vi "GetVarfromREPL.vi"(8 "error in (no error)":errorcluster, 10 "Command":string, 11 "Server":path) -> (0 "error out":errorcluster, 2 "reply":string)   [LabVIEW 2020]
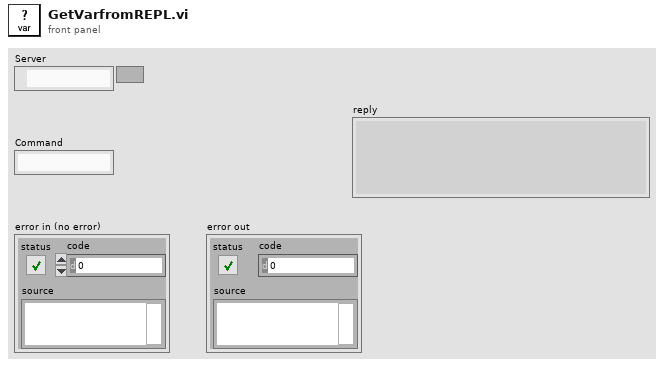
[diagram p1: front panel]
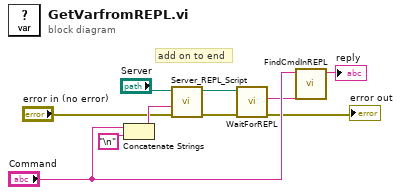
[diagram p0: block diagram]
diagram:
  # "add on to end"
  n1 = Concatenate Strings("Command", "\n") -> (w3:string)
  n2 = call "Server_REPL_Script.vi"("error in (no error)"="error in (no error)", "Code"=w3, "Server"="Server") -> ("error out"=w2:errorcluster)  [unwired: 8 in]
  n3 = call "WaitForREPL.vi"("error in (no error)"=w2, "Server"="Server") -> ("error out"=→"error out":errorcluster, "REPL"=w6:string)  [unwired: 8 in]
  n4 = call "FindCmdInREPL.vi"("File listing"=w6, "Command"="Command") -> ("reply"=→"reply":string)  [unwired: 9 in]
